vi "Generate Channels.vi"(8 "error in (no error)":errorcluster, 10 "Type":T2, 11 "Item Ref in":T6 format="%.0x") -> (0 "error out":errorcluster, 1 "Output Channels Out":T1[](array[typedef]), 2 "Input Channels Out":T1[](array[typedef]), 3 "Item Ref out":T6 format="%.0x")   [LabVIEW 2015, in "Modbus Master System Explorer.lvlib"]
uses:
  Modbus Master System Explorer.lvlib
  Shared/Controls/Data Model/Channel.ctl
  Modbus Type.ctl
  <vilib>/NI Veristand/Custom Device API/Custom Device Channel Type.ctl
  Shared/Controls/Data Model/Mapping.ctl
  Shared/Controls/Data Model/DataType.ctl
  <vilib>/NI Veristand/Custom Device API/Custom Device Item Ref.ctl
  <vilib>/NI Veristand/Custom Device Tools/Custom Device Utility Library/NI VeriStand - Search for Item by GUID.vi
  <vilib>/NI Veristand/Custom Device API/Get Item Property (U16).vi
  <vilib>/NI VeriStand/Custom Device Tools/Custom Device Utility Library/Custom Device Utility Library.lvlib
  Shared/Modbus Master Shared.lvlib
  <vilib>/NI VeriStand/Custom Device API/Custom Device API.lvlib
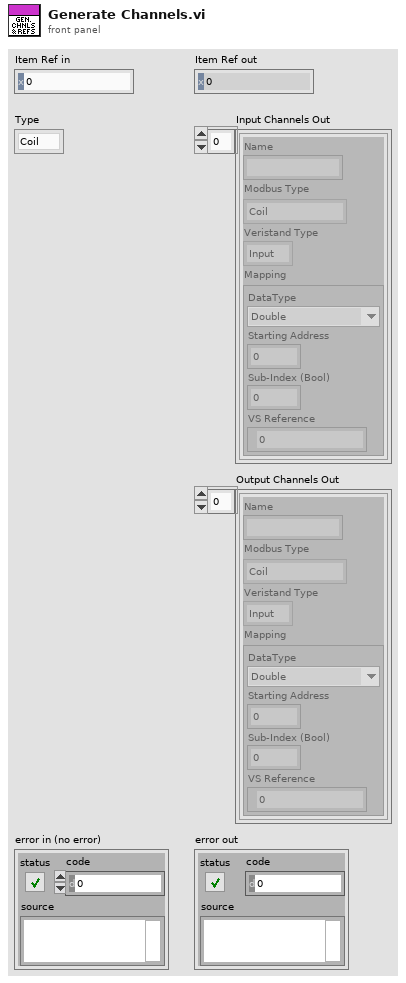
[diagram p1: front panel]
types:
  T1 = typedef "Modbus Master Shared.lvlib/Channel.ctl" = cluster{"Name":string, "Modbus Type":T2, "Veristand Type":T3, "Mapping":T4}
  T2 = typedef "Modbus Master Shared.lvlib/Modbus Type.ctl" = enum16{"Coil", "Discrete Input", "Holding Register", "Input Register"}
  T3 = typedef "Custom Device API.lvlib/Custom Device Channel Type.ctl" = enum16{"Input", "Output"}
  T4 = typedef "Modbus Master Shared.lvlib/Mapping.ctl" = cluster{"DataType":T5, "Starting Address":u16, "Sub-Index (Bool)":u16, "VS Reference":T6}
  T5 = typedef "Modbus Master Shared.lvlib/DataType.ctl" = enum16{"Double", "Single", "I64", "I32", "I16", "I8", "U64", "U32", "U16", "U8", "Boolean"}
  T6 = typedef "Custom Device API.lvlib/Custom Device Item Ref.ctl" = u64
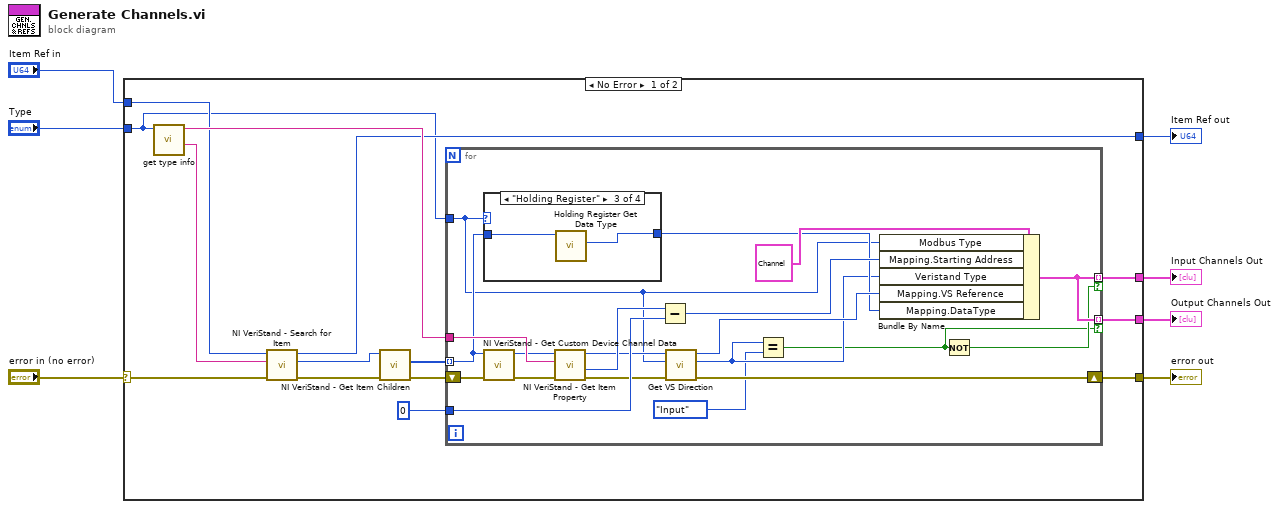
[diagram p0: block diagram]
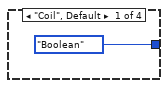
[diagram p2: hidden frame]
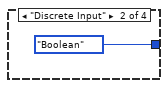
[diagram p3: hidden frame]
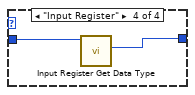
[diagram p4: hidden frame]
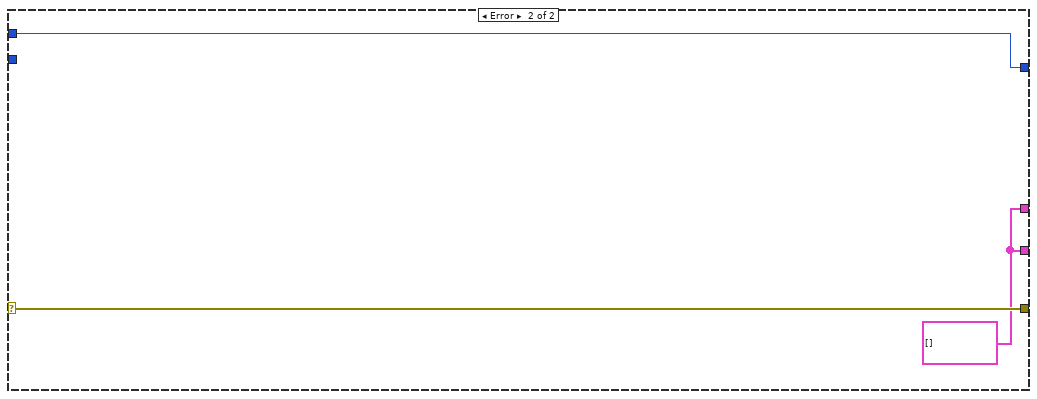
[diagram p5: hidden frame]
diagram:
  n1 = case shown="No Error" "error in (no error)" {
    selector: "error in (no error)" -> [w20 w49]
    tunnel: [w21 w49] -> w7
    tunnel: "Type" -> [w10 _]
    tunnel: "Item Ref in" -> [w18 w50]
    tunnel: [w11 w50] -> w3
    tunnel: [w17 w48] -> w2
    tunnel: [w8 w48] -> w1
    frame No Error {
      n2 = call "get type info.vi"("Type in"=w10) -> ("Group GUID"=w16:string, "Starting Address Tag"=w19:string)  [unwired: 7 in, 2 out]
      n3 = call-poly <vilib>:"NI VeriStand - Search for Item.vi"("error in"=w20, "Item GUID"=w16, "Section Ref in"=w18) -> ("error out"=w13:errorcluster, "Item Ref"=w15:T6, "Section Ref out"=w11:T6)  [unwired: 5 in, 1 out]
      n4 = call <vilib>:"NI VeriStand - Get Item Children.vi"("error in (no error)"=w13, "Item Ref in"=w15) -> ("error out"=w12:errorcluster, "Child Refs"=w14:T6[])  [unwired: 6 in, 2 out]
      n5 = for {
        tunnel: w14 -> [w28] mode=indexing
        tunnel: w19 -> [w40]
        tunnel: [w25] -> w17 mode=indexing if=w24
        shift-right: [w32] -> w21
        shift-left: w12 -> [w38]
        tunnel: u16 0 ("Offset") -> [w34]
        tunnel: w10 -> [w22]
        tunnel: [w25] -> w8 mode=indexing if=w23
        n6 = case shown="\"Holding Register\"" w22 {
          tunnel: [DataType."Boolean" ("Mapping.DataType") DataType."Boolean" ("Mapping.DataType") w44 w46] -> w29
          tunnel: w28 -> [_ _ w45 w47]
          frame "Coil", Default {
          }
          frame "Discrete Input" {
          }
          frame "Holding Register" {
            n7 = call "Holding Register Get Data Type.vi"("Item Ref in"=w45) -> ("Data Type"=w44:T5)  [unwired: 8 in, 2 out]
          }
          frame "Input Register" {
            n8 = call "Input Register Get Data Type.vi"("Item Ref in"=w47) -> ("Data Type"=w46:T5)  [unwired: 8 in, 2 out]
          }
        }
        n9 = call <vilib>:"NI VeriStand - Get Custom Device Channel Data.vi"("error in (no error)"=w38, "Channel Ref in"=w28) -> ("error out"=w37:errorcluster, "Channel Ref out"=w39:T6)  [unwired: 4 in, 4 out]
        n10 = call-poly <vilib>:"NI VeriStand - Get Item Property.vi"("error in (no error)"=w37, "Property Name"=w40, "Item Ref in"=w39) -> ("error out"=w33:errorcluster, "Value"=w36:u16, "Item Ref out"=w31:T6)  [unwired: 5 in, 1 out]
        n11 = Subtract(x=w36, y=w34) -> (x-y=w35:u16)
        n12 = call "Get VS Direction.vi"("error in (no error)"=w33, "Modbus Type"=w22, "Item Ref in"=w31) -> ("error out"=w32:errorcluster, "Veristand Type"=w27:T3, "Item Ref out"=w30:T6)  [unwired: 6 in]
        n13 = Equal?(x=w27, y=Custom_Device_Channel_Type."Input") -> (x = y?=w23:bool)
        n14 = Bundle By Name(cluster=T1 {"Name"="", "Modbus Type"=enum."Input Register", "Veristand Type"=enum."Input", "Mapping"={"DataType"=enum."Boolean", "Starting Address"=0, "Sub-Index (Bool)"=0, "VS Reference"=0}} ("Channel"), "Modbus Type"=w22, "Mapping.Starting Address"=w35, "Veristand Type"=w27, "Mapping.VS Reference"=w30, "Mapping.DataType"=w29) -> (w25:T1)
        n15 = Not(x=w23) -> (.not. x?=w24:bool)
      }
    }
    frame Error {
      w48 = T1[] []
    }
  }
  "error out" <- w7
  "Input Channels Out" <- w2
  "Item Ref out" <- w3
  "Output Channels Out" <- w1
